vi "Tones and Noise Waveform.vi"(4 "seed":i32=-1, 6 "sampling info":cluster{"Fs":dbl, "#s":dbl}={"Fs"=1000.0, "#s"=1000.0} {"Fs" format="%.2p"}, 7 "reset signal":bool, 8 "error in (no error)":errorcluster, 9 "offset":dbl format="%.2p", 10 "noise (rms)":dbl format="%.2p", 11 "tones":T1(array[cluster])=[{"frequency"=10.0, "amplitude"=1.0, "phase"=0.0}, {"frequency"=20.0, "amplitude"=0.1, "phase"=0.0}] {"phase" format="%.2p"; "amplitude" format="%0.2p"; "frequency" format="%0.2p"}) -> (0 "error out":errorcluster, 3 "signal out":waveform(dbl)={"t0"=timestamp(0.001 s since 1904-01-01), "dt"=1.0, "Y"=[]})   [LabVIEW 2020, in "NI_MABase.lvlib"]
doc: "Generates a waveform composed of a sum of sine tones, noise, and DC offset."
uses:
  NI_MABase.lvlib
  NI_AALBase.lvlib
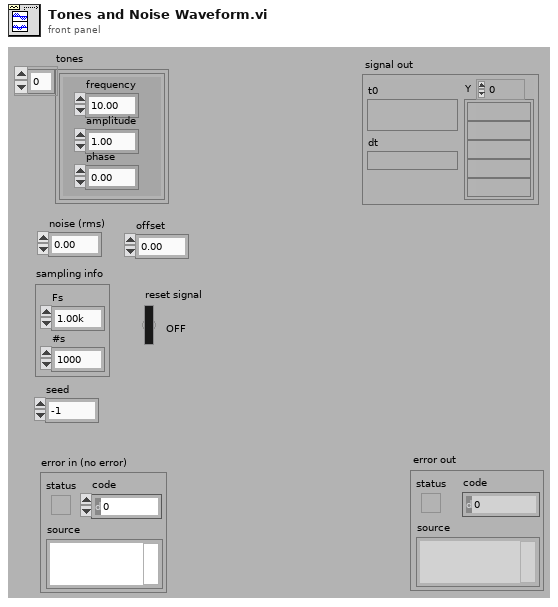
[diagram p1: front panel]
types:
  T1 = cluster{"frequency":dbl, "amplitude":dbl, "phase":dbl}[]
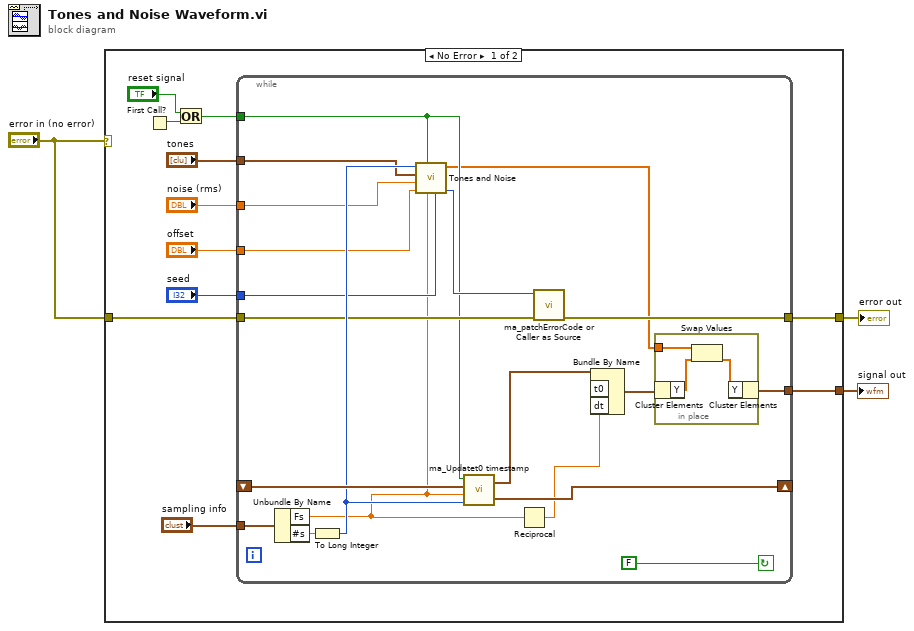
[diagram p0: block diagram]
diagram:
  n1 = case shown="No Error" "error in (no error)" {
    selector: "error in (no error)" -> [_ w38]
    tunnel: [w4 _] -> w2
    tunnel: [w12 w38] -> w3
    tunnel: "error in (no error)" -> [w8 _]
    frame No Error {
      n2 = First Call?() -> (First Call?: T/F=w7:bool)
      n3 = Or(x="reset signal", y=w7) -> (x .or. y?=w5:bool)
      n4 = while {
        tunnel: "sampling info" -> [w31]
        shift-left: _ -> [w34]
        shift-right: [w33] -> _
        tunnel: "tones" -> [w26]
        tunnel: [w29] -> w12
        tunnel: "seed" -> [w25]
        tunnel: w5 -> [w19]
        tunnel: "noise (rms)" -> [w23]
        tunnel: "offset" -> [w22]
        tunnel: w8 -> [w21]
        tunnel: [w16] -> w4
        stop <- FALSE continue-if-true
        n5 = Unbundle By Name(w31) -> ("Fs"=w15:dbl, "#s"=w30:dbl)
        n6 = To Long Integer(number=w30) -> (32bit integer=w27:i32)
        n7 = call "Tones and Noise.vi"("seed"=w25, "Fs"=w15, "reset signal"=w19, "offset"=w22, "noise (rms)"=w23, "tones"=w26, "samples"=w27) -> ("error"=w24:i32, "tones and noise"=w17:dbl[])  [unwired: 3 in]
        n8 = call "ma_Updatet0 timestamp.vi"("samples"=w27, "sampling rate (S/s)"=w15, "tf previous"=w34, "Reset Generation"=w19) -> ("tf new"=w33:timestamp, "t0"=w20:timestamp)
        n9 = Reciprocal(x=w15) -> (1/x=w28:dbl)
        n10 = call "ma_patchErrorCode or Caller as Source.vi"("error in (no error)"=w21, "error code"=w24) -> ("error out"=w29:errorcluster)  [unwired: 9 in]
        n11 = Bundle By Name("t0"=w20, "dt"=w28) -> (w18:waveform(dbl))  [unwired: 1 in]
        n12 = in-place {
          in-place-border: w17 -> [w36]
          n13 = in-place-cluster #1(w18) -> ("Y"=w37:dbl[])
          n14 = Swap Values(12:w36, 14:w37) -> (3:w35:dbl[])  [unwired: 1 in, 1 out]
          n15 = in-place-cluster #1("Y"=w35) -> (w16:waveform(dbl))
        }
      }
    }
    frame Error {
    }
  }
  "signal out" <- w2
  "error out" <- w3
